vi "update_temporal_calibration_locations.vi"(8 "error in (no error)":errorcluster, 11 "Projector to Camera Calibration in":T1) -> (0 "error out":errorcluster)   [LabVIEW 2019]
uses:
  <vilib>/vision/Image Controls.llb/IMAQ Image.ctl
  ParametersGlobal.vi
  <vilib>/vision/NI_Vision_Development_Module.lvlib
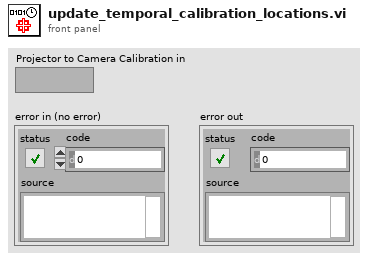
[diagram p1: front panel]
types:
  T1 = typedef "IMAQ Image.ctl" = refnum<image>
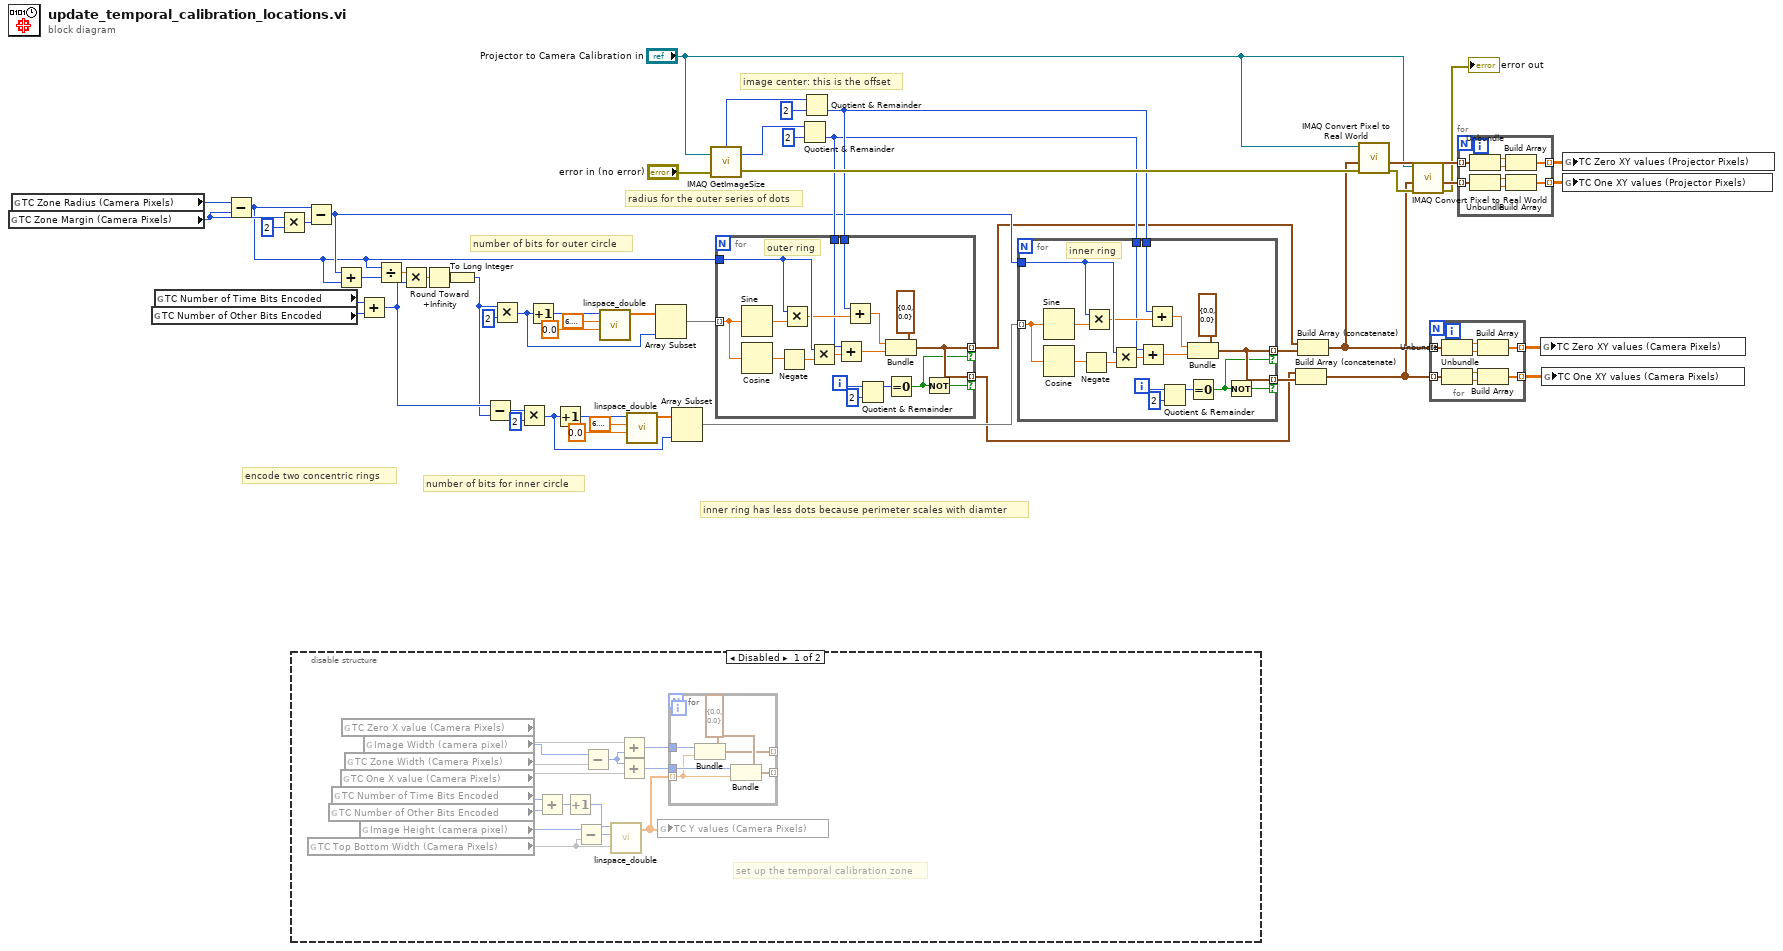
[diagram p0: block diagram]
diagram:
  # "number of bits for inner circle"
  # "inner ring has less dots because perimeter scales with diamter"
  # "number of bits for outer circle"
  # "encode two concentric rings"
  # "image center: this is the offset"
  # "radius for the outer series of dots"
  n1 = global read "ParametersGlobal.vi" "TC Zone Margin (Camera Pixels)"() -> (w25:i32)
  n2 = global read "ParametersGlobal.vi" "TC Zone Radius (Camera Pixels)"() -> (w49:i32)
  n3 = global read "ParametersGlobal.vi" "TC Number of Other Bits Encoded"() -> (w52:i32)
  n4 = global read "ParametersGlobal.vi" "TC Number of Time Bits Encoded"() -> (w51:i32)
  n5 = Subtract(x=w49, y=w25) -> (x-y=w20:i32)
  n6 = Multiply(x=w25, y=2) -> (x*y=w26:i32)
  n7 = disable-structure shown="Disabled" {
    frame Disabled {
      # "set up the temporal calibration zone"
      n8 = global read "ParametersGlobal.vi" "TC Top Bottom Width (Camera Pixels)"() -> (w59)
      n9 = global read "ParametersGlobal.vi" "TC Number of Other Bits Encoded"() -> (w56:i32)
      n10 = global read "ParametersGlobal.vi" "TC Number of Time Bits Encoded"() -> (w57:i32)
      n11 = global read "ParametersGlobal.vi" "TC One X value (Camera Pixels)"() -> (w66)
      n12 = global read "ParametersGlobal.vi" "TC Zero X value (Camera Pixels)"() -> (w67)
      n13 = global read "ParametersGlobal.vi" "TC Zone Width (Camera Pixels)"() -> (w65)
      n14 = global read "ParametersGlobal.vi" "Image Height (camera pixel)"() -> (w58:i32)
      n15 = global read "ParametersGlobal.vi" "Image Width (camera pixel)"() -> (w64:i32)
      n16 = Add(x=w57, y=w56) -> (x+y=w55:i32)
      n17 = Increment(x=w55) -> (x+1=w54:i32)
      n18 = Subtract(x=w58, y=w59) -> (x-y=w53:i32)
      n19 = Subtract(x=w64, y=w65) -> (x-y=w60:i32)
      n20 = call "linspace_double.vi"("start"=w59, "end"=w53, "samples"=w54) -> ("Ramp Pattern"=w63:dbl[])  [unwired: 8 in]
      n21 = Add(x=w67, y=w60) -> (x+y=w61:i32)
      n22 = Add(x=w60, y=w66) -> (x+y=w62:i32)
      n23 = global write "ParametersGlobal.vi" "TC Y values (Camera Pixels)"(w63) -> ()
      n24 = for {
        tunnel: w61 -> [w72]
        tunnel: w62 -> [w71]
        tunnel: w63 -> [w70] mode=indexing
        tunnel: [w69] -> _ mode=indexing
        tunnel: [w68] -> _ mode=indexing
        w73 = cluster{"X":sgl, "Y":sgl} {"X"=0.0, "Y"=0.0} ("Camera Point")
        n25 = Bundle(cluster=w73, "X"=w72, "Y"=w70) -> (w69:cluster{"X":sgl, "Y":sgl})
        n26 = Bundle(cluster=w73, "X"=w71, "Y"=w70) -> (w68:cluster{"X":sgl, "Y":sgl})
      }
    }
    frame Enabled {
    }
  }
  n27 = Subtract(x=w20, y=w26) -> (x-y=w23:i32)
  n28 = Add(x=w23, y=w20) -> (x+y=w21:i32)
  n29 = Add(x=w51, y=w52) -> (x+y=w17:i32)
  n30 = Divide(x=w20, y=w21) -> (x/y=w19:dbl)
  n31 = Multiply(x=w19, y=w17) -> (x*y=w18:dbl)
  n32 = Round Toward +Infinity(x=w18) -> (ceil(x): smallest int >= x=w16:dbl)
  n33 = To Long Integer(number=w16) -> (32bit integer=w15:i32)
  n34 = Subtract(x=w17, y=w15) -> (x-y=w9:i32)
  n35 = Multiply(x=w15, y=2) -> (x*y=w45:i32)
  n36 = Multiply(x=w9, y=2) -> (x*y=w8:i32)
  n37 = Increment(x=w45) -> (x+1=w48:i32)
  n38 = Increment(x=w8) -> (x+1=w13:i32)
  n39 = call "linspace_double.vi"("start"=0.0, "end"=6.283185307179586, "samples"=w48) -> ("Ramp Pattern"=w46:dbl[])  [unwired: 8 in]
  n40 = call "linspace_double.vi"("start"=0.0, "end"=6.283185307179586, "samples"=w13) -> ("Ramp Pattern"=w11:dbl[])  [unwired: 8 in]
  n41 = Array Subset(array=w46, length=w45) -> (w44:dbl[])  [unwired: 1 in]
  n42 = Array Subset(array=w11, length=w8) -> (w7:dbl[])  [unwired: 1 in]
  n43 = call "IMAQ GetImageSize"("Image"="Projector to Camera Calibration in", "error in (no error)"="error in (no error)") -> ("Y Resolution"=w35:i32, "X Resolution"=w34:i32, "error out"=w33:errorcluster)  [unwired: 2 in]
  n44 = Quotient & Remainder(x=w35, y=2) -> (floor(x/y)=w27:i32)  [unwired: 1 out]
  n45 = Quotient & Remainder(x=w34, y=2) -> (floor(x/y)=w28:i32)  [unwired: 1 out]
  n46 = for {
    tunnel: [w84] -> w6 mode=indexing if=w82
    tunnel: w44 -> [w87] mode=indexing
    tunnel: w20 -> [w85]
    tunnel: [w84] -> w3 mode=indexing if=w83
    tunnel: w27 -> [w77]
    tunnel: w28 -> [w76]
    i -> [w90]
    # "outer ring"
    n47 = Sine(x=w87) -> (sin(x)=w86:dbl)
    n48 = Cosine(x=w87) -> (cos(x)=w81:dbl)
    n49 = Negate(x=w81) -> (-x=w80:dbl)
    n50 = Multiply(x=w85, y=w86) -> (x*y=w79:dbl)
    n51 = Multiply(x=w85, y=w80) -> (x*y=w78:dbl)
    n52 = Add(x=w77, y=w78) -> (x+y=w74:dbl)
    n53 = Add(x=w76, y=w79) -> (x+y=w75:dbl)
    n54 = Quotient & Remainder(x=w90, y=2) -> (x-y*floor(x/y)=w88:i32)  [unwired: 1 out]
    n55 = Bundle(cluster=cluster{"X":sgl, "Y":sgl} {"X"=0.0, "Y"=0.0} ("Camera Point"), "X"=w75, "Y"=w74) -> (w84:cluster{"X":sgl, "Y":sgl})
    n56 = Equal To 0?(x=w88) -> (x = 0?=w82:bool)
    n57 = Not(x=w82) -> (.not. x?=w83:bool)
  }
  n58 = for {
    tunnel: [w102] -> w5 mode=indexing if=w100
    tunnel: w7 -> [w105] mode=indexing
    tunnel: w23 -> [w103]
    tunnel: [w102] -> w4 mode=indexing if=w101
    tunnel: w27 -> [w95]
    tunnel: w28 -> [w94]
    i -> [w108]
    # "inner ring"
    n59 = Sine(x=w105) -> (sin(x)=w104:dbl)
    n60 = Cosine(x=w105) -> (cos(x)=w99:dbl)
    n61 = Negate(x=w99) -> (-x=w98:dbl)
    n62 = Multiply(x=w103, y=w104) -> (x*y=w97:dbl)
    n63 = Multiply(x=w103, y=w98) -> (x*y=w96:dbl)
    n64 = Add(x=w95, y=w96) -> (x+y=w92:dbl)
    n65 = Add(x=w94, y=w97) -> (x+y=w93:dbl)
    n66 = Quotient & Remainder(x=w108, y=2) -> (x-y*floor(x/y)=w106:i32)  [unwired: 1 out]
    n67 = Bundle(cluster=cluster{"X":sgl, "Y":sgl} {"X"=0.0, "Y"=0.0} ("Camera Point"), "X"=w93, "Y"=w92) -> (w102:cluster{"X":sgl, "Y":sgl})
    n68 = Equal To 0?(x=w106) -> (x = 0?=w100:bool)
    n69 = Not(x=w100) -> (.not. x?=w101:bool)
  }
  n70 = Build Array (concatenate)(w3, w4) -> (w1:cluster{"X":sgl, "Y":sgl}[])
  n71 = Build Array (concatenate)(w6, w5) -> (w2:cluster{"X":sgl, "Y":sgl}[])
  n72 = call "IMAQ Convert Pixel to Real World"("error in (no error)"=w33, "Array of Pixel Coordinates"=w2, "Calibrated Image"="Projector to Camera Calibration in") -> ("error out"=w41:errorcluster, "Array of Real World Coordinates"=w39:cluster{"X":sgl, "Y":sgl}[])  [unwired: 3 in, 4 out]
  n73 = call "IMAQ Convert Pixel to Real World"("error in (no error)"=w41, "Array of Pixel Coordinates"=w1, "Calibrated Image"="Projector to Camera Calibration in") -> ("error out"=→"error out":errorcluster, "Array of Real World Coordinates"=w40:cluster{"X":sgl, "Y":sgl}[])  [unwired: 3 in, 4 out]
  n74 = for {
    tunnel: w2 -> [w117] mode=indexing
    tunnel: w1 -> [w112] mode=indexing
    tunnel: [w111] -> w29 mode=indexing
    tunnel: [w110] -> w30 mode=indexing
    n75 = Unbundle(w117) -> ("X"=w116:sgl, "Y"=w115:sgl)
    n76 = Unbundle(w112) -> ("X"=w114:sgl, "Y"=w113:sgl)
    n77 = Build Array(w116, w115) -> (w111:sgl[])
    n78 = Build Array(w114, w113) -> (w110:sgl[])
  }
  n79 = for {
    tunnel: w39 -> [w125] mode=indexing
    tunnel: w40 -> [w120] mode=indexing
    tunnel: [w119] -> w43 mode=indexing
    tunnel: [w118] -> w42 mode=indexing
    n80 = Unbundle(w125) -> ("X"=w124:sgl, "Y"=w123:sgl)
    n81 = Unbundle(w120) -> ("X"=w122:sgl, "Y"=w121:sgl)
    n82 = Build Array(w124, w123) -> (w119:sgl[])
    n83 = Build Array(w122, w121) -> (w118:sgl[])
  }
  n84 = global write "ParametersGlobal.vi" "TC Zero XY values (Camera Pixels)"(w29) -> ()
  n85 = global write "ParametersGlobal.vi" "TC One XY values (Camera Pixels)"(w30) -> ()
  n86 = global write "ParametersGlobal.vi" "TC Zero XY values (Projector Pixels)"(w43) -> ()
  n87 = global write "ParametersGlobal.vi" "TC One XY values (Projector Pixels)"(w42) -> ()
